vi "smooth.vi"(1 "length":i32, 2 "Array in":dbl[](array[numeric]) format="%.2f") -> (0 "Array out":dbl[](array[numeric]) format="%.2f")   [LabVIEW 2013]
uses:
  <vilib>/Analysis/baseanly.llb/Mean (DBL).vi
  <vilib>/Analysis/NI_AALBase.lvlib
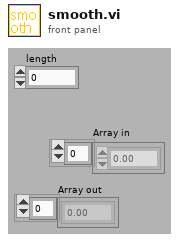
[diagram p1: front panel]
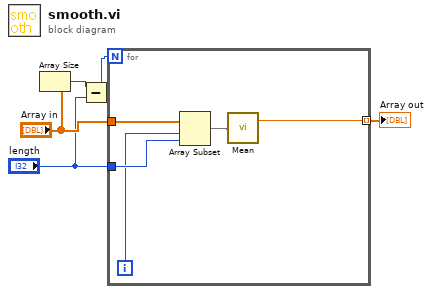
[diagram p0: block diagram]
diagram:
  n1 = Array Size(array="Array in") -> (size(s)=w2:i32)
  n2 = Subtract(x=w2, y="length") -> (x-y=w3:i32)
  n3 = for {
    N: w3 -> [_]
    tunnel: "Array in" -> [w9]
    tunnel: "length" -> [w10]
    tunnel: [w6] -> w1 mode=indexing
    i -> [w8]
    n4 = Array Subset(array=w9, index=w8, length=w10) -> (w7:dbl[])
    n5 = call-poly <vilib>:"Mean.vi"("X"=w7) -> ("mean"=w6:dbl)  [unwired: 1 out]
  }
  "Array out" <- w1
